vi "Macro Action String to Action and Settings Enum.vi"(8 "error in (no error)":errorcluster, 11 "Action String IN":string) -> (0 "error out":errorcluster, 1 "Settings File Type OUT (String)":string, 2 "Setting File Type OUT":T1=enum."Configuration Settings", 3 "Action Enum OUT":T2)   [LabVIEW 2012]
doc: "SciScan 1.2 160622"
uses:
  MacroGUI Module/Custom Controls and Typedefs/Macro_Action_List.ctl
  Custom Controls/Setting File Types.ctl
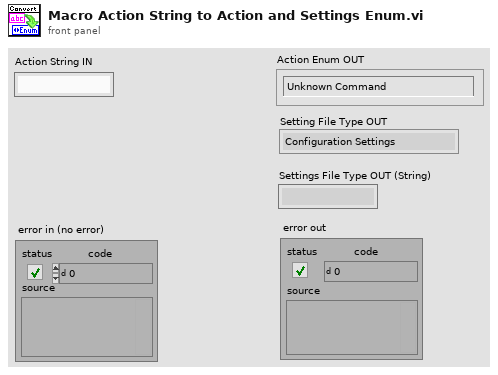
[diagram p1: front panel]
types:
  T1 = typedef "Setting File Types.ctl" = enum16{"2D.Frame.Scan.Settings", "2D.Line.Scan.Settings", "Z.Stack.Settings", "HW Settings", "Configuration Settings", "Unknown Settings", "Fast.Z.Settings"}
  T2 = typedef "Macro_Action_List.ctl" = enum16{"Unknown Command", "2D.Frame.Scan", "2D.Line.Scan", "Load.Settings.File", "Move.To.Position", "Pause", "Z.Stack", "LOOP.Start", "LOOP.End", "Record", "Fast.Z", "Generic", "Slow.Z", "Tiling", "Preset.End"}
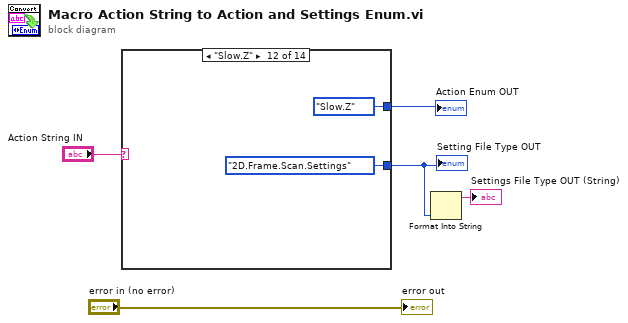
[diagram p0: block diagram]
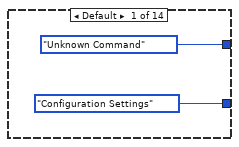
[diagram p2: hidden frame]
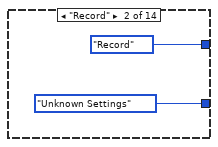
[diagram p3: hidden frame]
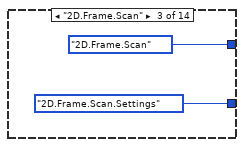
[diagram p4: hidden frame]
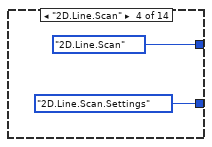
[diagram p5: hidden frame]
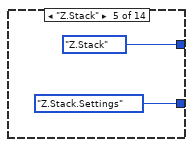
[diagram p6: hidden frame]
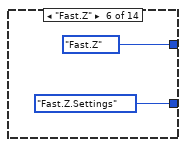
[diagram p7: hidden frame]
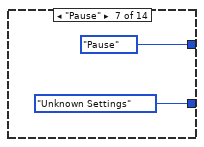
[diagram p8: hidden frame]
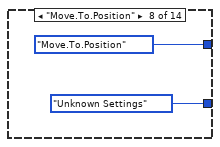
[diagram p9: hidden frame]
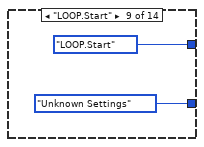
[diagram p10: hidden frame]
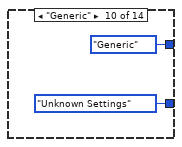
[diagram p11: hidden frame]
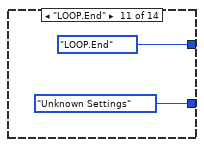
[diagram p12: hidden frame]
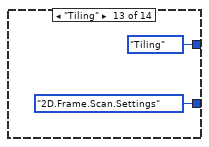
[diagram p13: hidden frame]
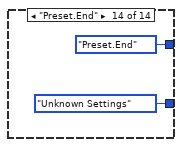
[diagram p14: hidden frame]
diagram:
  n1 = case shown="\"Slow.Z\"" "Action String IN" {
    tunnel: [Macro_Action_List."Unknown Command" ("Action Enum OUT") Macro_Action_List."Record" ("Action Enum OUT") Macro_Action_List."2D.Frame.Scan" ("Action Enum OUT") Macro_Action_List."2D.Line.Scan" ("Action Enum OUT") Macro_Action_List."Z.Stack" ("Action Enum OUT") Macro_Action_List."Fast.Z" ("Action Enum OUT") Macro_Action_List."Pause" ("Action Enum OUT") Macro_Action_List."Move.To.Position" ("Action Enum OUT") Macro_Action_List."LOOP.Start" ("Action Enum OUT") Macro_Action_List."Generic" ("Action Enum OUT") Macro_Action_List."LOOP.End" ("Action Enum OUT") Macro_Action_List."Slow.Z" ("Action Enum OUT") Macro_Action_List."Tiling" ("Action Enum OUT") Macro_Action_List."Preset.End" ("Action Enum OUT")] -> w4
    tunnel: [Setting_File_Types."Configuration Settings" ("Setting File Type OUT") Setting_File_Types."Unknown Settings" ("Setting File Type OUT") Setting_File_Types."2D.Frame.Scan.Settings" ("Setting File Type OUT") Setting_File_Types."2D.Line.Scan.Settings" ("Setting File Type OUT") Setting_File_Types."Z.Stack.Settings" ("Setting File Type OUT") Setting_File_Types."Fast.Z.Settings" ("Setting File Type OUT") Setting_File_Types."Unknown Settings" ("Setting File Type OUT") Setting_File_Types."Unknown Settings" ("Setting File Type OUT") Setting_File_Types."Unknown Settings" ("Setting File Type OUT") Setting_File_Types."Unknown Settings" ("Setting File Type OUT") Setting_File_Types."Unknown Settings" ("Setting File Type OUT") Setting_File_Types."2D.Frame.Scan.Settings" ("Setting File Type OUT") Setting_File_Types."2D.Frame.Scan.Settings" ("Setting File Type OUT") Setting_File_Types."Unknown Settings" ("Setting File Type OUT")] -> w2
    frame Default {
    }
    frame "Record" {
    }
    frame "2D.Frame.Scan" {
    }
    frame "2D.Line.Scan" {
    }
    frame "Z.Stack" {
    }
    frame "Fast.Z" {
    }
    frame "Pause" {
    }
    frame "Move.To.Position" {
    }
    frame "LOOP.Start" {
    }
    frame "Generic" {
    }
    frame "LOOP.End" {
    }
    frame "Slow.Z" {
    }
    frame "Tiling" {
    }
    frame "Preset.End" {
    }
  }
  "Action Enum OUT" <- w4
  "Setting File Type OUT" <- w2
  n2 = Format Into String(w2) -> (resulting string=→"Settings File Type OUT (String)":string)  [unwired: 3 in, 1 out]
  "error out" <- "error in (no error)"
